vi "Acquire Signals.vi"(8 "error in (no error)":errorcluster, 11 "Connected?":bool[](array[boolean])) -> (0 "error out":errorcluster, 3 "Array":dbl[][](array[numeric]))   [LabVIEW 2020]
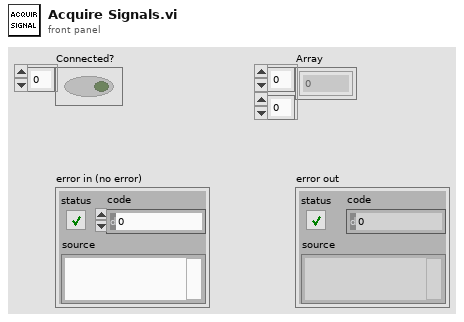
[diagram p1: front panel]
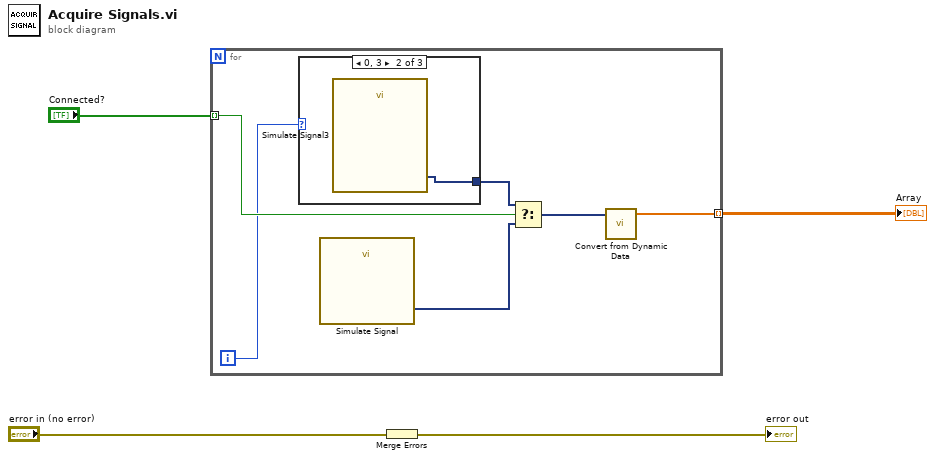
[diagram p0: block diagram]
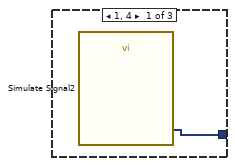
[diagram p2: hidden frame]
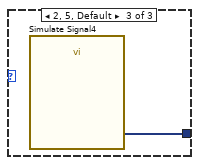
[diagram p3: hidden frame]
diagram:
  n1 = for {
    tunnel: "Connected?" -> [w8] mode=indexing
    tunnel: [w6] -> w3 mode=indexing
    i -> [w5]
    n2 = case shown="0, 3" w5 {
      tunnel: [w11 w12 w13] -> w10
      frame 1, 4 {
        n3 = call "Simulate Signal2"() -> ("Triangle with Uniform Noise"=w11:dynamicdata)  [unwired: 14 in, 1 out]
      }
      frame 0, 3 {
        n4 = call "Simulate Signal3"() -> ("Sine with Uniform Noise"=w12:dynamicdata)  [unwired: 14 in, 1 out]
      }
      frame 2, 5, Default {
        n5 = call "Simulate Signal4"() -> ("Sawtooth with Uniform Noise"=w13:dynamicdata)  [unwired: 14 in, 1 out]
      }
    }
    n6 = call "Simulate Signal"() -> ("DC with Uniform Noise"=w9:dynamicdata)  [unwired: 14 in, 1 out]
    n7 = Select(t=w10, s=w8, f=w9) -> (s? t:f=w7:dynamicdata)
    n8 = call "Convert from Dynamic Data"("Dynamic Data Type"=w7) -> ("Array"=w6:dbl[])  [unwired: 3 in]
  }
  "Array" <- w3
  n9 = Merge Errors("error in (no error)") -> (→"error out":errorcluster)
